vi "Call Bootloader on COM Device.vi"(0 "port":refnum<visa-resource-name>, 11 "error in (no error)":errorcluster) -> (4 "port out":refnum<visa-resource-name>, 15 "error out":errorcluster)   [LabVIEW 2010]
uses:
  <vilib>/Instr/_visa.llb/VISA Flush IO Buffer Mask.ctl
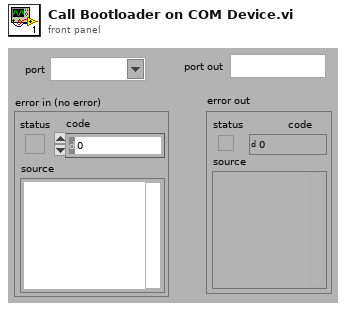
[diagram p1: front panel]
types:
  T1 = typedef "VISA Flush IO Buffer Mask.ctl" = u16
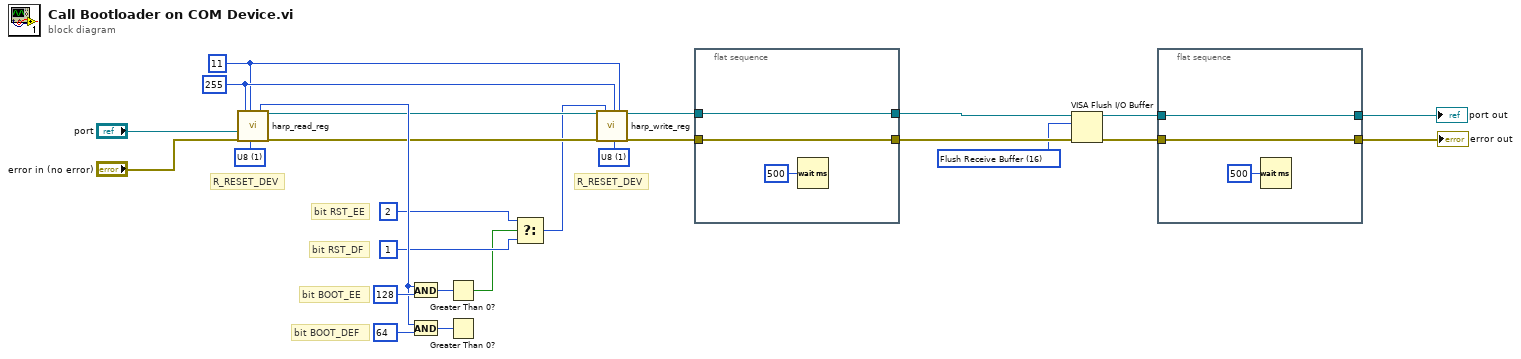
[diagram p0: block diagram]
diagram:
  w5 = T1 16 items=["Flush Receive Buffer"=16, "Write Transmit Buffer to Device"=32, "Flush Receive Buffer (No I/O)"=64, "Flush Transmit Buffer"=128] ("Mask")
  w10 = u8 1 items=["U8"=1, "U16"=2, "U32"=4, "U64"=8, "I8"=129, "I16"=130, "I32"=132, "I64"=136, "FLOAT"=68, "BOOL"=17] ("type")
  w11 = u8 11 ("reg. address")
  w12 = u8 255 ("port")
  w26 = u8 1 items=["U8"=1, "U16"=2, "U32"=4, "U64"=8, "I8"=129, "I16"=130, "I32"=132, "I64"=136, "FLOAT"=68, "BOOL"=17] ("type")
  # "R_RESET_DEV"
  # "bit RST_DF"
  # "bit RST_EE"
  # "bit BOOT_DEF"
  # "bit BOOT_EE"
  # "R_RESET_DEV"
  n1 = call "harp_read_reg.vi"(0:"port"="port", "error in (no error)"="error in (no error)", 6:"port"=w12, "reg. address"=w11, "type"=w26) -> ("8 bits"=w21:u8, "port out"=w14:refnum<visa-resource-name>, "error out"=w15:errorcluster)  [unwired: 5 in, 7 out]
  n2 = And(x=w21, y=u8 128) -> (x .and. y?=w20:u8)
  n3 = And(x=w21, y=u8 64) -> (x .and. y?=w19:u8)
  n4 = Greater Than 0?(x=w20) -> (x > 0?=w16:bool)
  n5 = Greater Than 0?(x=w19) -> ()  [unwired: 1 out]
  n6 = Select(t=u8 2 ("y"), s=w16, f=u8 1 ("y")) -> (s? t:f=w13:u8)
  n7 = call "harp_write_reg.vi"(0:"port"=w14, "error in (no error)"=w15, "8 bits"=w13, 10:"port"=w12, "type"=w10, "reg. address"=w11) -> ("port out"=w8:refnum<visa-resource-name>, "error out"=w9:errorcluster)  [unwired: 11 in, 1 out]
  n8 = flat-sequence {
    tunnel: [w29] -> w7
    tunnel: w9 -> [w29]
    tunnel: [w28] -> w6
    tunnel: w8 -> [w28]
    frame #0 {
      n9 = Wait (ms)(milliseconds to wait=u32 500) -> ()  [unwired: 1 out]
    }
  }
  n10 = VISA Flush I/O Buffer(VISA resource name=w6, mask (16)=w5, error in (no error)=w7) -> (VISA resource name out=w3:refnum<visa-resource-name>, error out=w4:errorcluster)
  n11 = flat-sequence {
    tunnel: [w32] -> w1
    tunnel: w4 -> [w32]
    tunnel: [w31] -> w2
    tunnel: w3 -> [w31]
    frame #0 {
      n12 = Wait (ms)(milliseconds to wait=u32 500) -> ()  [unwired: 1 out]
    }
  }
  "error out" <- w1
  "port out" <- w2
